vi "FS Body Cylinder.vi"(8 "Body #":i32=1, 9 "Cylinder":T1={"Point 1"={"x"=0.0, "y"=0.0, "z"=0.0}, "Point 2"={"x"=1.0, "y"=1.0, "z"=1.0}, "Radius"=1.0}, 11 "Feature In":string="FeatureScript 1247;\nimport(path : \"onshape/std/geometry.fs\", version : \"1247.0\");\n\nannotation { \"Feature Type Name\" : \"LabVIEW Feature\" }\nexport const myFeature = defineFeature(function(context is Context, id is Id, definition is map)\n    precondition\n    {\n        // Define the parameters of the feature type\n    }\n    {\n        // Define the function's action\n    });") -> (3 "Feature Out":string="FeatureScript 1247;\nimport(path : \"onshape/std/geometry.fs\", version : \"1247.0\");\n\nannotation { \"Feature Type Name\" : \"LVFeat1\" }\nexport const myFeature = defineFeature(function(context is Context, id is Id, definition is map)\n    precondition\n    {\n        // Define the parameters of the feature type\n    }\n    {\n        // Define the function's action\n       fEllipsoid(context, id + \"ellipsoid1\", {\n                \"center\" : vector(5, 0, 0) * inch,\n                \"radius\" : vector(3, 3, 3) * inch,\n        });\n\nvar sketch1 = newSketch(context, id + \"sketch1\", {\n                \"sketchPlane\" : qCreatedBy(makeId(\"Top\"), EntityType.FACE)\n        });\n        // Create sketch entities here\n        skRectangle(sketch1, \"rectangle1\", {\n                \"firstCorner\" : vector(0, 0) * inch,\n                \"secondCorner\" : vector(3, 4) * inch\n        });\n        \n        skSolve(sketch1);\n    });")   [LabVIEW 2019]
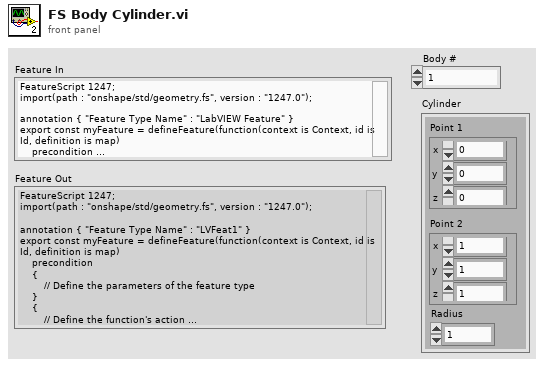
[diagram p1: front panel]
types:
  T1 = cluster{"Point 1":cluster{"x":dbl, "y":dbl, "z":dbl}, "Point 2":cluster{"x":dbl, "y":dbl, "z":dbl}, "Radius":dbl}
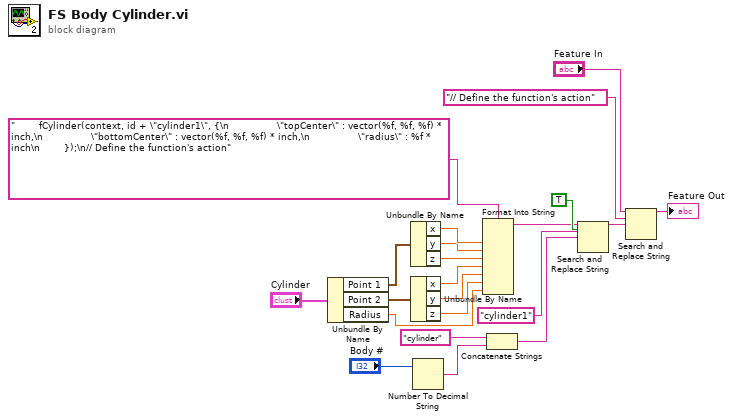
[diagram p0: block diagram]
diagram:
  n1 = Unbundle By Name("Cylinder") -> ("Point 1"=w20:cluster{"x":dbl, "y":dbl, "z":dbl}, "Point 2"=w21:cluster{"x":dbl, "y":dbl, "z":dbl}, "Radius"=w3:dbl)
  n2 = Unbundle By Name(w20) -> ("x"=w9:dbl, "y"=w8:dbl, "z"=w7:dbl)
  n3 = Unbundle By Name(w21) -> ("x"=w6:dbl, "y"=w5:dbl, "z"=w4:dbl)
  n4 = Number To Decimal String(number="Body #") -> (decimal integer string=w14:string)  [unwired: 1 in]
  n5 = Format Into String(format string="        fCylinder(context, id + \"cylinder1\", {\n                \"topCenter\" : vector(%f, %f, %f) * inch,\n                \"bottomCenter\" : vector(%f, %f, %f) * inch,\n                \"radius\" : %f * inch\n        });\n// Define the function's action" ("search string"), w9, w8, w7, w6, w5, w4, w3) -> (resulting string=w2:string)  [unwired: 2 in, 1 out]
  n6 = Concatenate Strings("cylinder" ("regular expression"), w14) -> (w18:string)
  n7 = Search and Replace String(replace all?=TRUE ("replace all? (F)"), input string=w2, search string="cylinder1" ("regular expression"), replace string=w18) -> (result string=w10:string)  [unwired: 4 in, 3 out]
  n8 = Search and Replace String(input string="Feature In", search string="// Define the function's action", replace string=w10) -> (result string=→"Feature Out":string)  [unwired: 5 in, 3 out]
